vi "Test Circular Subarray.vi"() -> ()   [LabVIEW 2015]
uses:
  Math VIs/LinSpace (x0-dx-npts).vi
panel:
  out "Waveform Graph":dbl[](graph)
  in  "Offset":i32
  in  "Num Subarrays":i32=1
  in  "Npts/subarray":i32=20
  in  "Array Length":i32=100
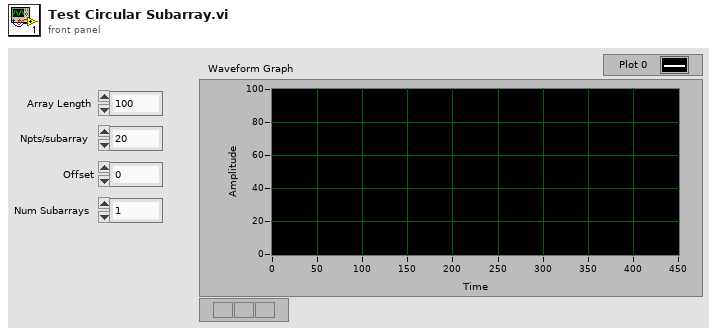
[diagram p1: front panel]
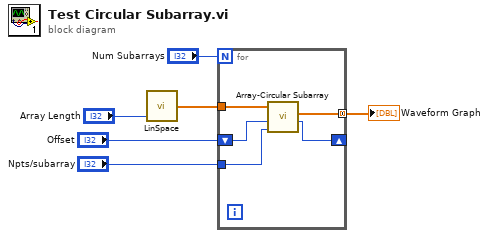
[diagram p0: block diagram]
diagram:
  n1 = call-poly "LinSpace.vi"("npts"="Array Length") -> ("Array"=w4:dbl[])  [unwired: 3 in, 1 out]
  n2 = for {
    N: "Num Subarrays" -> [_]
    tunnel: w4 -> [w11]
    shift-right: [w9] -> _
    shift-left: "Offset" -> [w10]
    tunnel: [w8] -> w1 mode=concatenating
    tunnel: "Npts/subarray" -> [w7]
    n3 = call "Array-Circular Subarray.vi"("Npts"=w7, "Offset (in)"=w10, "Array"=w11) -> ("Offset (out)"=w9:i32, "Subarray"=w8:dbl[])  [unwired: 7 in]
  }
  "Waveform Graph" <- w1
